vi "CAN-SET.vi"(6 "DevIndex":u32, 9 "open?":bool, 10 "type":u32(ring)=2 items=["USB-CAN"=2, "USB-CAN2.0"=3]) -> (2 "success":bool, 3 "Param out":T2[](array[typedef]) {"ACR0" format="%x"})   [LabVIEW 2011]
doc: "ID=0x6000"
uses:
  VIs/Param.ctl
  VIs/Baud rate Self Define.ctl
  VIs/ParamType.ctl
panel:
  out "label3":string="注：CAN波特率=16000000/(同步段+传播时间段+相位缓冲段1+相位缓冲段2)/预分频"
  out "label4":string="滤波器"
  out "label1":string="工作模式"
  out "label2":string="波特率设置"
  in  "advance":bool
  in  "br_selfdef":T1={"BAUD"=0, "SJW"=1, "BRP"=1, "SAM"=0, "PHS2_SEL"=0, "SYN(nouse)"=1, "PRSEG"=1, "PHSEG1"=1, "PHSEG2"=1} {"PHSEG2" items=["CAN_BIT_1TQ"=1, "CAN_BIT_2TQ"=2, "CAN_BIT_3TQ"=3, "CAN_BIT_4TQ"=4, "CAN_BIT_5TQ"=5, "CAN_BIT_6TQ"=6, "CAN_BIT_7TQ"=7, "CAN_BIT_8TQ"=8]; "PHSEG1" items=["CAN_BIT_1TQ"=1, "CAN_BIT_2TQ"=2, "CAN_BIT_3TQ"=3, "CAN_BIT_4TQ"=4, "CAN_BIT_5TQ"=5, "CAN_BIT_6TQ"=6, "CAN_BIT_7TQ"=7, "CAN_BIT_8TQ"=8]; "PRSEG" items=["CAN_BIT_1TQ"=1, "CAN_BIT_2TQ"=2, "CAN_BIT_3TQ"=3, "CAN_BIT_4TQ"=4, "CAN_BIT_5TQ"=5, "CAN_BIT_6TQ"=6, "CAN_BIT_7TQ"=7, "CAN_BIT_8TQ"=8]; "PHS2_SEL" items=["由相位缓冲段1时间指定", "可编程"]; "SAM" items=["采样一次", "采样三次"]; "BRP" items=["1"=1, "2"=2, "3"=3, "4"=4, "5"=5, "6"=6, "7"=7, "8"=8, "9"=9, "10"=10, "11"=11, "12"=12, "13"=13, "14"=14, "15"=15, "16"=16, "17"=17, "18"=18, "19"=19, "20"=20, "21"=21, "22"=22, "23"=23, "24"=24, "25"=25, "26"=26, "27"=27, "28"=28, "29"=29, "30"=30, "31"=31, "32"=32, "33"=33, "34"=34, "35"=35, "36"=36, "37"=37, "38"=38, "39"=39, "40"=40, "41"=41, "42"=42, "43"=43, "44"=44, "45"=45, "46"=46, "47"=47, "48"=48, "49"=49, "50"=50, "51"=51, "52"=52, "53"=53, "54"=54, "55"=55, "56"=56, "57"=57, "58"=58, "59"=59, "60"=60, "61"=61, "62"=62, "63"=63, "64"=64]; "SJW" items=["1TQ"=1, "2TQ"=2, "3TQ"=3, "4TQ"=4]; "SYN(nouse)" items=["CAN_BIT_1TQ"=1]}
  in  "Filter":u8(ring)=1 caption="滤波方式:" items=["接收所有类型"=1, "只收标准帧"=2, "只收扩展帧"=3]
  in  "set2":bool
  in  "set1":bool
  in  "channel":u16(ring) caption="CAN通道:" items=["通道1", "通道2"]
  in  "屏蔽码":u32=4294967295 caption="过滤屏蔽码:" format="%08x"
  in  "验收码":u32=2147483648 caption="过滤验收码:" format="%08x"
  in  "工作模式":u16(ring) items=["正常工作", "监听(只听)", "自发自收(环回/自测)", "正常工作并接收错误帧"]
  in  "set0":bool
  in  "br":u32(ring)=8 caption="波特率:" items=["Self Define", "5k bps", "10k bps", "20k bps", "40k bps", "50k bps", "80k bps", "100k bps", "125k bps", "200k bps", "250k bps", "400k bps", "500k bps", "666k bps", "800k bps", "1000k bps", "33.33k bps", "66.66k bps", "83.33k bps"]
  # "(HEX)"
  # "(HEX)"
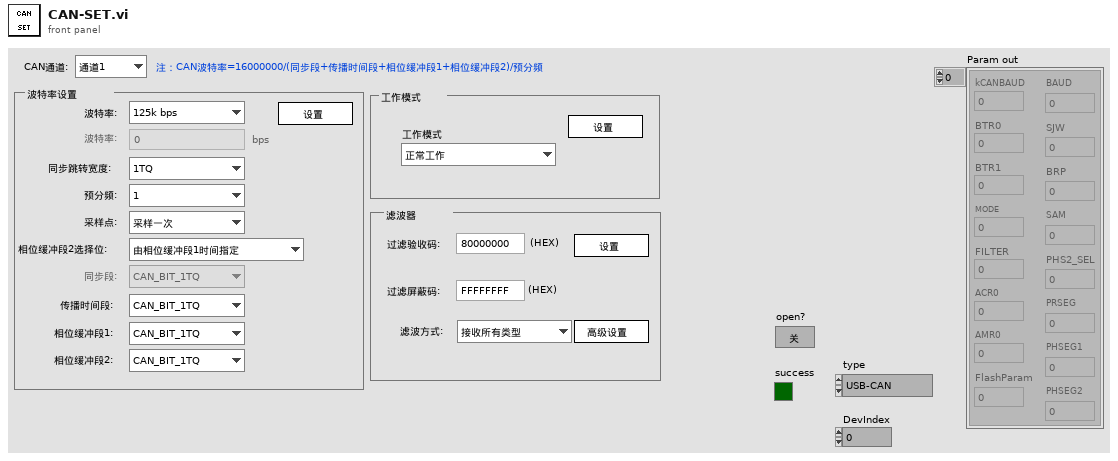
[diagram p1: front panel]
types:
  T1 = typedef "Baud rate Self Define.ctl" = cluster{"BAUD":u32, "SJW":u8, "BRP":u8, "SAM":u8, "PHS2_SEL":u8, "SYN(nouse)":u8, "PRSEG":u8, "PHSEG1":u8, "PHSEG2":u8}
  T2 = typedef "Param.ctl" = cluster{"kCANBAUD":u8, "BTR0":u8, "BTR1":u8, "MODE":u8, "FILTER":u8, "ACR0":u32, "AMR0":u32, "FlashParam":u32, "BAUD":u32, "SJW":u8, "BRP":u8, "SAM":u8, "PHS2_SEL":u8, "PRSEG":u8, "PHSEG1":u8, "PHSEG2":u8}
  T3 = enum8{"Enabled", "Disabled", "Disabled and Grayed Out"}
  T4 = typedef "ParamType.ctl" = u32
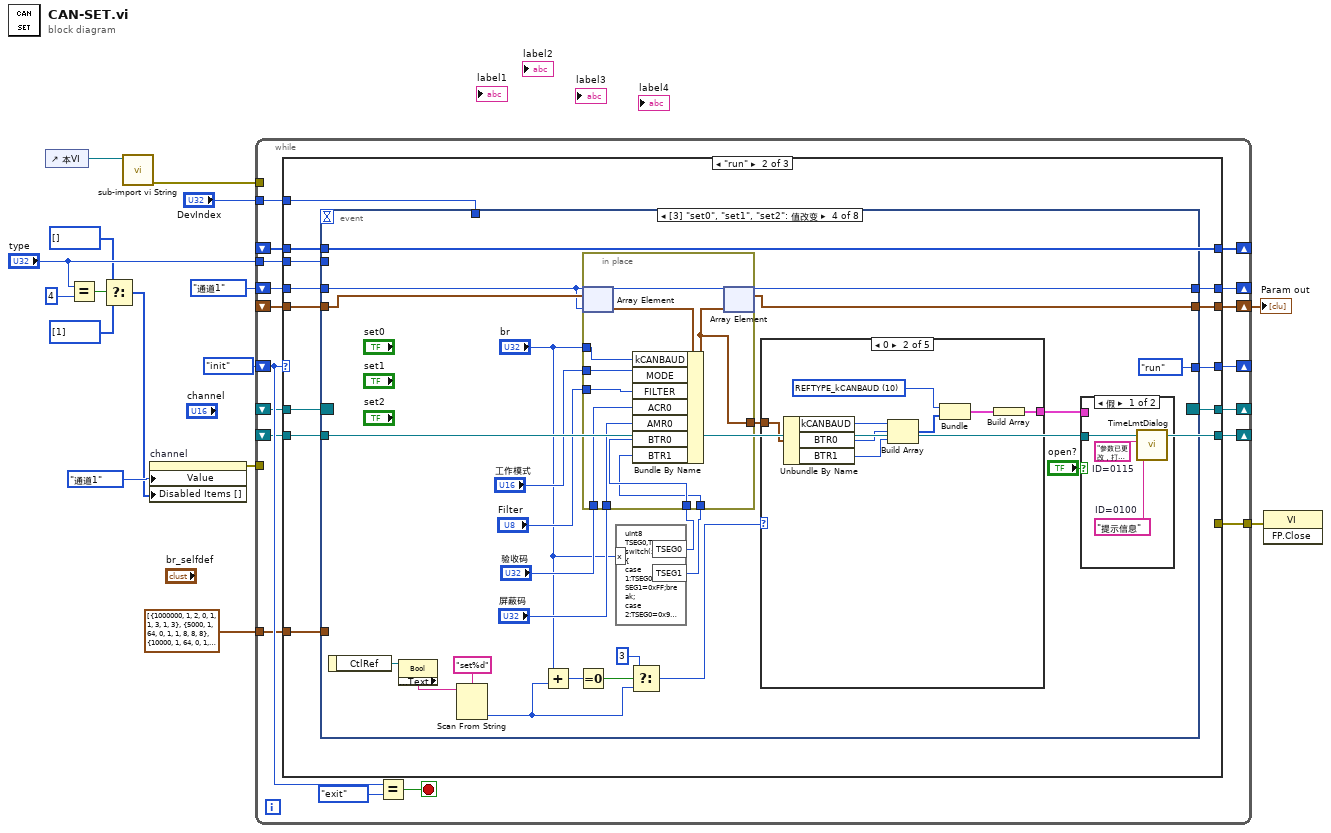
[diagram p0: block diagram]
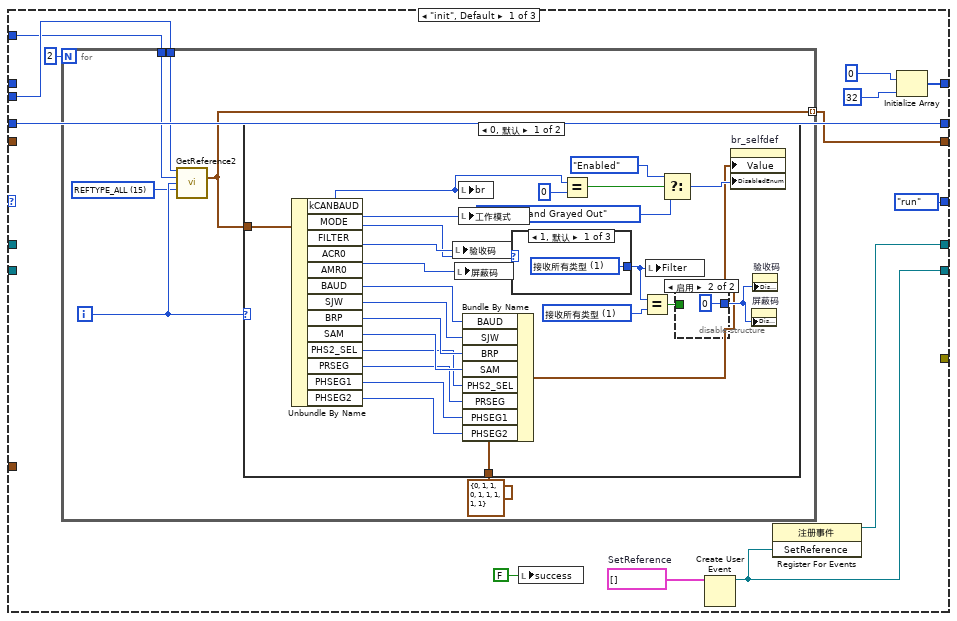
[diagram p2: hidden frame]
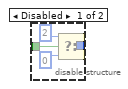
[diagram p3: hidden frame]
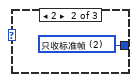
[diagram p4: hidden frame]
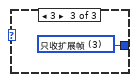
[diagram p5: hidden frame]
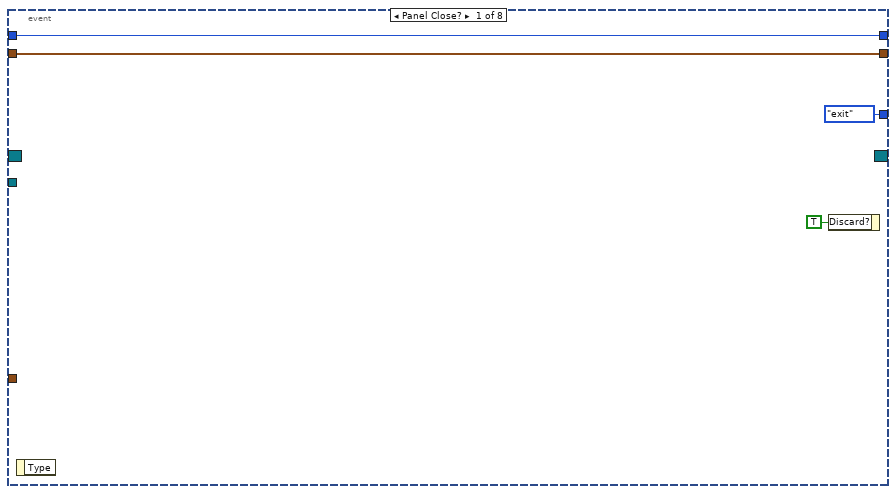
[diagram p7: hidden frame]
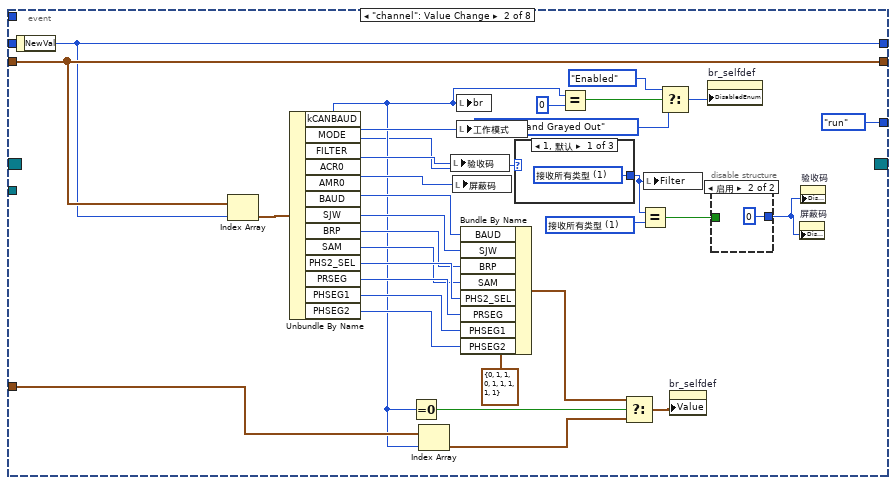
[diagram p8: hidden frame]
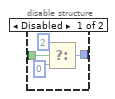
[diagram p9: hidden frame]
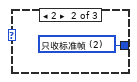
[diagram p10: hidden frame]
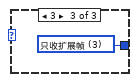
[diagram p11: hidden frame]
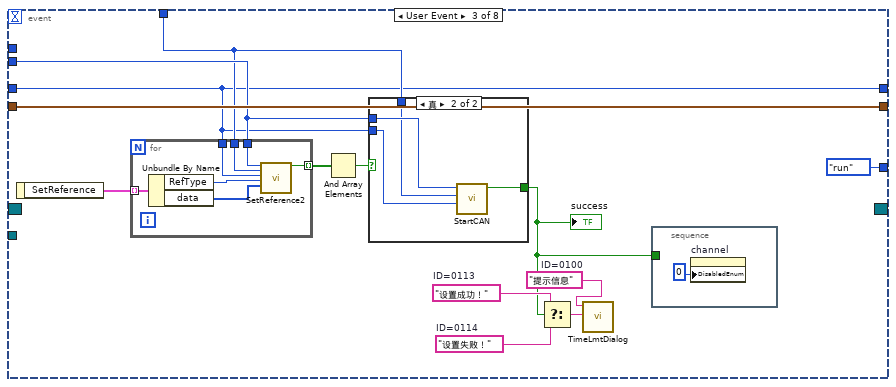
[diagram p12: hidden frame]
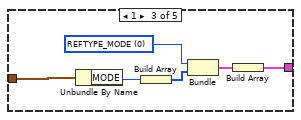
[diagram p15: hidden frame]
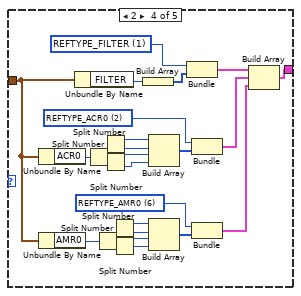
[diagram p16: hidden frame]
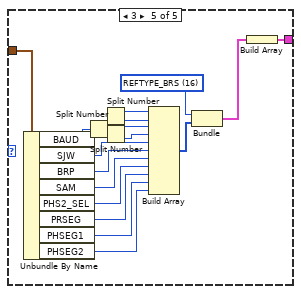
[diagram p17: hidden frame]
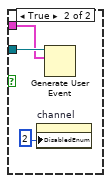
[diagram p18: hidden frame]
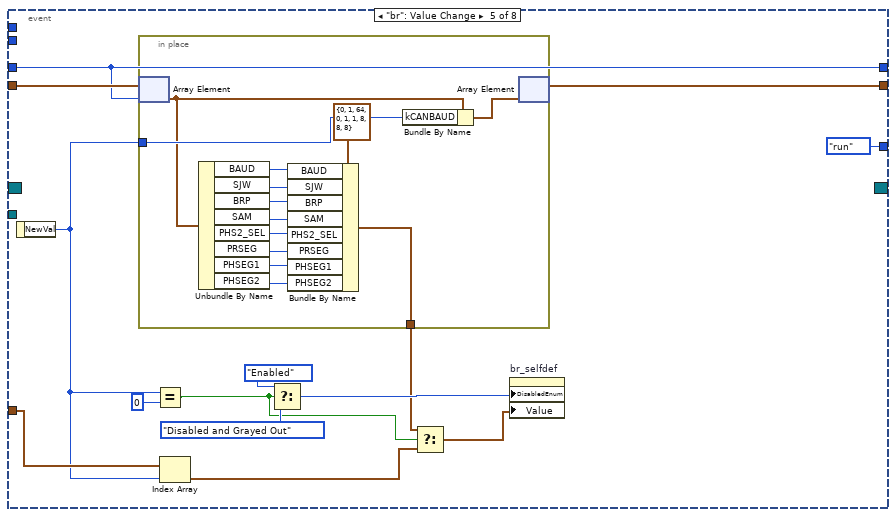
[diagram p19: hidden frame]
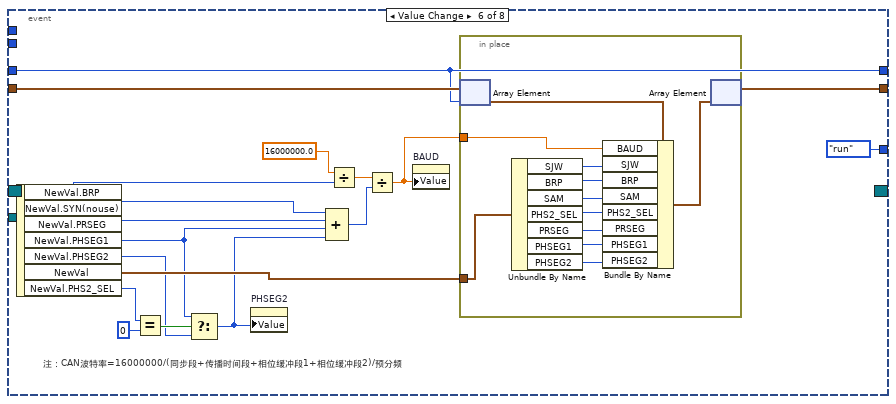
[diagram p20: hidden frame]
diagram:
  n1 = control-ref of="本VI"() -> (w2:refnum<vi>)
  n2 = Equal?(x="type", y=u32 4) -> (x = y?=w9:bool)
  n3 = Select(t=i32[] [] ("禁用项[]"), s=w9, f=i32[] [1] ("禁用项[]")) -> (s? t:f=w7:i32[])
  n4 = call "sub-import vi String.vi"("vi ref"=w2) -> ("error out"=w1:errorcluster)  [unwired: 10 in]
  n5 = property on="channel" class="Ring (严格)"("Value"=enum16{"通道1", "通道2"}."通道1" ("channel"), "Disabled Items []"=w7) -> (error out=w14:errorcluster)  [unwired: 2 in, 1 out]
  n6 = while {
    shift-right: [w33] -> w4
    shift-left: _ -> [w34]
    shift-right: [w32] -> _
    shift-left: enum16{"init", "run", "exit"}."init" -> [w31]
    tunnel: [w28] -> w15
    shift-right: [w27] -> _
    shift-left: _ -> [w25]
    shift-right: [w26] -> _
    shift-left: _ -> [w24]
    tunnel: "type" -> [w23]
    shift-right: [w22] -> _
    shift-left: _ -> [w21]
    tunnel: "DevIndex" -> [w20]
    shift-right: [w18] -> _
    shift-left: enum16{"通道1", "通道2"}."通道1" ("NewVal") -> [w19]
    tunnel: w14 -> [_]
    tunnel: T1[] [{"BAUD"=1000000, "SJW"=1, "BRP"=2, "SAM"=0, "PHS2_SEL"=1, "SYN(nouse)"=1, "PRSEG"=3, "PHSEG1"=1, "PHSEG2"=3}, {"BAUD"=5000, "SJW"=1, "BRP"=64, "SAM"=0, "PHS2_SEL"=1, "SYN(nouse)"=1, "PRSEG"=8, "PHSEG1"=8, "PHSEG2"=8}, {"BAUD"=10000, "SJW"=1, "BRP"=64, "SAM"=0, "PHS2_SEL"=1, "SYN(nouse)"=1, "PRSEG"=8, "PHSEG1"=8, "PHSEG2"=8}, {"BAUD"=20000, "SJW"=1, "BRP"=50, "SAM"=0, "PHS2_SEL"=1, "SYN(nouse)"=1, "PRSEG"=5, "PHSEG1"=5, "PHSEG2"=5}, {"BAUD"=40000, "SJW"=1, "BRP"=16, "SAM"=0, "PHS2_SEL"=1, "SYN(nouse)"=1, "PRSEG"=8, "PHSEG1"=8, "PHSEG2"=8}, {"BAUD"=50000, "SJW"=1, "BRP"=20, "SAM"=0, "PHS2_SEL"=1, "SYN(nouse)"=1, "PRSEG"=5, "PHSEG1"=5, "PHSEG2"=5}, {"BAUD"=80000, "SJW"=1, "BRP"=8, "SAM"=0, "PHS2_SEL"=1, "SYN(nouse)"=1, "PRSEG"=8, "PHSEG1"=8, "PHSEG2"=8}, {"BAUD"=100000, "SJW"=1, "BRP"=10, "SAM"=0, "PHS2_SEL"=1, "SYN(nouse)"=1, "PRSEG"=7, "PHSEG1"=4, "PHSEG2"=4}, {"BAUD"=125000, "SJW"=1, "BRP"=8, "SAM"=0, "PHS2_SEL"=1, "SYN(nouse)"=1, "PRSEG"=7, "PHSEG1"=4, "PHSEG2"=4}, {"BAUD"=200000, "SJW"=1, "BRP"=4, "SAM"=0, "PHS2_SEL"=1, "SYN(nouse)"=1, "PRSEG"=7, "PHSEG1"=6, "PHSEG2"=6}, {"BAUD"=250000, "SJW"=1, "BRP"=4, "SAM"=0, "PHS2_SEL"=1, "SYN(nouse)"=1, "PRSEG"=7, "PHSEG1"=4, "PHSEG2"=4}, {"BAUD"=400000, "SJW"=1, "BRP"=2, "SAM"=0, "PHS2_SEL"=1, "SYN(nouse)"=1, "PRSEG"=7, "PHSEG1"=6, "PHSEG2"=6}, {"BAUD"=500000, "SJW"=1, "BRP"=2, "SAM"=0, "PHS2_SEL"=1, "SYN(nouse)"=1, "PRSEG"=7, "PHSEG1"=4, "PHSEG2"=4}, {"BAUD"=666000, "SJW"=1, "BRP"=2, "SAM"=0, "PHS2_SEL"=1, "SYN(nouse)"=1, "PRSEG"=3, "PHSEG1"=4, "PHSEG2"=4}, {"BAUD"=800000, "SJW"=1, "BRP"=2, "SAM"=0, "PHS2_SEL"=1, "SYN(nouse)"=1, "PRSEG"=3, "PHSEG1"=3, "PHSEG2"=3}, {"BAUD"=1000000, "SJW"=1, "BRP"=2, "SAM"=0, "PHS2_SEL"=1, "SYN(nouse)"=1, "PRSEG"=3, "PHSEG1"=1, "PHSEG2"=3}, {"BAUD"=33333, "SJW"=1, "BRP"=32, "SAM"=0, "PHS2_SEL"=1, "SYN(nouse)"=1, "PRSEG"=4, "PHSEG1"=5, "PHSEG2"=5}, {"BAUD"=66666, "SJW"=1, "BRP"=16, "SAM"=0, "PHS2_SEL"=1, "SYN(nouse)"=1, "PRSEG"=4, "PHSEG1"=5, "PHSEG2"=5}, {"BAUD"=83333, "SJW"=1, "BRP"=8, "SAM"=0, "PHS2_SEL"=1, "SYN(nouse)"=1, "PRSEG"=7, "PHSEG1"=8, "PHSEG2"=8}] -> [w17]
    tunnel: w1 -> [_]
    stop <- w29 stop-if-true
    n7 = case shown="\"run\"" w31 {
      tunnel: w34 -> [_ w98 w370]
      tunnel: [w37 w97 w370] -> w33
      tunnel: [enum16{"init", "run", "exit"}."run" w96 enum16{"init", "run", "exit"}."exit"] -> w32
      tunnel: [_ _ errorcluster {"status"=FALSE, "code"=0, "source"=""} ("错误输入（无错误）")] -> w28
      tunnel: [w46 w91 _] -> w27
      tunnel: [w45 w92 _] -> w26
      tunnel: w25 -> [_ w95 w367]
      tunnel: w24 -> [_ w92 w365]
      tunnel: w23 -> [w36 w94 _]
      tunnel: [w42 w93 _] -> w22
      tunnel: w21 -> [_ w93 _]
      tunnel: w20 -> [w35 w90 _]
      tunnel: w19 -> [w39 w89 w364]
      tunnel: [w39 w88 w364] -> w18
      tunnel: w17 -> [_ w87 _]
      frame "init", Default {
        w40 = cluster{"RefType":u32, "data":u8[]}[] []  # SetReference
        n8 = for {
          N: 2 -> [_]
          tunnel: [w48] -> w37 mode=indexing
          tunnel: w36 -> [w52]
          tunnel: w35 -> [w51]
          i -> [w53]
          w50 = T4 15 items=["REFTYPE_MODE"=0, "REFTYPE_FILTER"=1, "REFTYPE_ACR0"=2, "REFTYPE_AMR0"=6, "REFTYPE_kCANBAUD"=10, "REFTYPE_CANRX_EN"=13, "REFTYPE_UARTBAUD"=14, "REFTYPE_ALL"=15, "REFTYPE_BRS"=16] ("RefType")
          n9 = call "GetReference2.vi"("DeviceType"=w52, "DeviceInd"=w51, "CANInd"=w53, "RefType"=w50) -> ("Param"=w48:T2)  [unwired: 9 in, 2 out]
          n10 = case shown="0, 默认" w53 {
            tunnel: w48 -> [w72 _]
            tunnel: T1 {"BAUD"=0, "SJW"=1, "BRP"=1, "SAM"=0, "PHS2_SEL"=1, "SYN(nouse)"=1, "PRSEG"=1, "PHSEG1"=1, "PHSEG2"=1} ("br_selfdef") -> [w69 _]
            frame 0, Default {
              w55 = u8 1 items=["接收所有类型"=1, "只收标准帧"=2, "只收扩展帧"=3] ("Filter")
              n11 = Unbundle By Name(w72) -> ("kCANBAUD"=w58:u8, "MODE"=w78:u8, "FILTER"=w56:u8, "ACR0"=w77:u32, "AMR0"=w76:u32, "BAUD"=w67:u32, "SJW"=w66:u8, "BRP"=w65:u8, "SAM"=w64:u8, "PHS2_SEL"=w63:u8, "PRSEG"=w62:u8, "PHSEG1"=w61:u8, "PHSEG2"=w60:u8)
              n12 = local write "验收码"(w77) -> ()
              n13 = local write "屏蔽码"(w76) -> ()
              n14 = local write "br"(w58) -> ()
              n15 = local write "工作模式"(w78) -> ()
              n16 = Bundle By Name(cluster=w69, "BAUD"=w67, "SJW"=w66, "BRP"=w65, "SAM"=w64, "PHS2_SEL"=w63, "PRSEG"=w62, "PHSEG1"=w61, "PHSEG2"=w60) -> (w57:T1)
              n17 = case shown="1, 默认" w56 {
                tunnel: [w84 w85 w86] -> w54
                frame 1, Default {
                  w84 = u8 1 items=["接收所有类型"=1, "只收标准帧"=2, "只收扩展帧"=3] ("Filter")
                }
                frame 2 {
                  w85 = u8 2 items=["接收所有类型"=1, "只收标准帧"=2, "只收扩展帧"=3] ("Filter")
                }
                frame 3 {
                  w86 = u8 3 items=["接收所有类型"=1, "只收标准帧"=2, "只收扩展帧"=3] ("Filter")
                }
              }
              n18 = Equal?(x=w58, y=u32 0) -> (x = y?=w59:bool)
              n19 = Equal?(x=w54, y=w55) -> (x = y?=w71:bool)
              n20 = local write "Filter"(w54) -> ()
              n21 = Select(t=T3."Enabled" ("禁用"), s=w59, f=T3."Disabled and Grayed Out") -> (s? t:f=w68:T3)
              n22 = disable-structure shown="启用" {
                disable-tunnel: w71 -> [w82 _]
                disable-tunnel: [w81 0] -> w70
                frame Disabled {
                  n23 = Select(t=2, s=w82, f=0) -> (s? t:f=w81:i32)
                }
                frame Enabled {
                }
              }
              n24 = property on="br_selfdef" class="Clust (严格)"("Value"=w57, "DisabledEnum"=w68) -> ()  [unwired: 2 in, 2 out]
              n25 = property on="屏蔽码" class="DigNum (严格)"("DisabledEnum"=w70) -> ()  [unwired: 2 in, 2 out]
              n26 = property on="验收码" class="DigNum (严格)"("DisabledEnum"=w70) -> ()  [unwired: 2 in, 2 out]
            }
            frame 1 {
            }
          }
        }
        n27 = local write "success"(FALSE ("success")) -> ()
        n28 = Create User Event(user event datatype=w40) -> (user event=w45:refnum<user-event>)  [unwired: 1 in, 1 out]
        n29 = register-events(w45) -> (reference out=w46:refnum<event-registration>)  [unwired: 2 in, 1 out]
        n30 = Initialize Array(u8 0, 32 ("维数大小")) -> (w42:u8[])
      }
      frame "run" {
        n31 = event shown="[3] \"set0\", \"set1\", \"set2\": 值改变" {
          selector: w95 -> [_ _ _ _ _ _ _ _]
          dyn-events: [_ _ _ _ _ _ _ _] -> w91
          timeout: _ -> [_ _ _ _ _ _ _ _]
          tunnel: w98 -> [w101 w133 w155 w180 w273 w302 w323 w355]
          tunnel: [w101 w133 w155 w178 w272 w300 w321 w355] -> w97
          tunnel: [enum16{"init", "run", "exit"}."exit" enum16{"init", "run", "exit"}."run" enum16{"init", "run", "exit"}."run" enum16{"init", "run", "exit"}."run" enum16{"init", "run", "exit"}."run" enum16{"init", "run", "exit"}."run" enum16{"init", "run", "exit"}."run" enum16{"init", "run", "exit"}."run"] -> w96
          tunnel: w92 -> [_ _ _ w189 _ _ _ _]
          tunnel: w94 -> [_ _ w149 _ _ _ _ _]
          tunnel: w93 -> [_ _ _ _ _ _ _ _]
          tunnel: w90 -> [_ _ w148 _ _ _ _ _]
          tunnel: w89 -> [w99 _ w145 w179 w267 w301 w322 w358]
          tunnel: [w99 w132 w145 w179 w267 w301 w322 w358] -> w88
          tunnel: w87 -> [_ w108 _ _ w268 _ _ _]
          event Panel Close? {
            n32 = event-data() -> ()  [unwired: 1 in, 1 out]
            n33 = event-data("Discard?"=TRUE ("放弃？")) -> ()  [unwired: 1 in, 1 out]
          }
          event "channel": Value Change {
            w103 = u8 1 items=["接收所有类型"=1, "只收标准帧"=2, "只收扩展帧"=3] ("Filter")
            n34 = event-data() -> ("NewVal"=w132:u16)  [unwired: 1 in]
            n35 = Index Array(array=w133, index=w132) -> (element=w112:T2)
            n36 = Unbundle By Name(w112) -> ("kCANBAUD"=w107:u8, "MODE"=w114:u8, "FILTER"=w105:u8, "ACR0"=w115:u32, "AMR0"=w116:u32, "BAUD"=w123:u32, "SJW"=w124:u8, "BRP"=w125:u8, "SAM"=w126:u8, "PHS2_SEL"=w127:u8, "PRSEG"=w128:u8, "PHSEG1"=w129:u8, "PHSEG2"=w130:u8)
            n37 = Equal To 0?(x=w107) -> (x = 0?=w111:bool)
            n38 = Index Array(array=w108, index=w107) -> (element=w106:T1)
            n39 = local write "验收码"(w115) -> ()
            n40 = local write "屏蔽码"(w116) -> ()
            n41 = local write "br"(w107) -> ()
            n42 = local write "工作模式"(w114) -> ()
            n43 = Bundle By Name(cluster=T1 {"BAUD"=0, "SJW"=1, "BRP"=1, "SAM"=0, "PHS2_SEL"=1, "SYN(nouse)"=1, "PRSEG"=1, "PHSEG1"=1, "PHSEG2"=1} ("br_selfdef"), "BAUD"=w123, "SJW"=w124, "BRP"=w125, "SAM"=w126, "PHS2_SEL"=w127, "PRSEG"=w128, "PHSEG1"=w129, "PHSEG2"=w130) -> (w110:T1)
            n44 = case shown="1, 默认" w105 {
              tunnel: [w140 w141 w142] -> w104
              frame 1, Default {
                w140 = u8 1 items=["接收所有类型"=1, "只收标准帧"=2, "只收扩展帧"=3] ("Filter")
              }
              frame 2 {
                w141 = u8 2 items=["接收所有类型"=1, "只收标准帧"=2, "只收扩展帧"=3] ("Filter")
              }
              frame 3 {
                w142 = u8 3 items=["接收所有类型"=1, "只收标准帧"=2, "只收扩展帧"=3] ("Filter")
              }
            }
            n45 = Equal?(x=w107, y=u32 0) -> (x = y?=w131:bool)
            n46 = Select(t=w110, s=w111, f=w106) -> (s? t:f=w109:T1)
            n47 = Equal?(x=w104, y=w103) -> (x = y?=w120:bool)
            n48 = local write "Filter"(w104) -> ()
            n49 = Select(t=T3."Enabled" ("禁用"), s=w131, f=T3."Disabled and Grayed Out") -> (s? t:f=w122:T3)
            n50 = property on="br_selfdef" class="Clust (严格)"("Value"=w109) -> ()  [unwired: 2 in, 2 out]
            n51 = property on="br_selfdef" class="Clust (严格)"("DisabledEnum"=w122) -> ()  [unwired: 2 in, 2 out]
            n52 = disable-structure shown="启用" {
              disable-tunnel: [w136 0] -> w121
              disable-tunnel: w120 -> [w135 _]
              frame Disabled {
                n53 = Select(t=2, s=w135, f=0) -> (s? t:f=w136:i32)
              }
              frame Enabled {
              }
            }
            n54 = property on="屏蔽码" class="DigNum (严格)"("DisabledEnum"=w121) -> ()  [unwired: 2 in, 2 out]
            n55 = property on="验收码" class="DigNum (严格)"("DisabledEnum"=w121) -> ()  [unwired: 2 in, 2 out]
          }
          event User Event {
            w143 = "提示信息"  # ID=0100
            w152 = "设置失败！"  # ID=0114
            w153 = "设置成功！"  # ID=0113
            n56 = event-data() -> ("SetReference"=w147:cluster{"RefType":u32, "data":u8[]}[])  [unwired: 1 in]
            n57 = for {
              tunnel: [w163] -> w150 mode=indexing
              tunnel: w149 -> [w162]
              tunnel: w148 -> [w161]
              tunnel: w145 -> [w160]
              tunnel: w147 -> [w159] mode=indexing
              n58 = Unbundle By Name(w159) -> ("RefType"=w158:u32, "data"=w157:u8[])
              n59 = call "SetReference2.vi"("DeviceType"=w162, "DeviceInd"=w161, "CANInd"=w160, "RefType"=w158, "pData"=w157) -> ("Success"=w163:bool)  [unwired: 13 in, 1 out]
            }
            n60 = And Array Elements(Boolean array=w150) -> (logical AND=w146:bool)
            n61 = case shown="真" w146 {
              tunnel: w149 -> [_ w167]
              tunnel: w145 -> [_ w165]
              tunnel: [_ w164] -> w144
              tunnel: w148 -> [_ w166]
              frame False {
              }
              frame True {
                n62 = call "StartCAN.vi"("CANInd"=w165, "DeciceInd"=w166, "DeviceType"=w167) -> ("Valid"=w164:bool)  [unwired: 7 in, 1 out]
              }
            }
            "success" <- w144
            n63 = Select(t=w153, s=w144, f=w152) -> (s? t:f=w151:string)
            n64 = call "TimeLmtDialog.vi"("Infoin"=w151, "title"=w143) -> ()  [unwired: 10 in]
            n65 = stacked-sequence {
              tunnel: w144 -> [_]
              frame #0 {
                n66 = property on="channel" class="Ring (严格)"("DisabledEnum"=0) -> ()  [unwired: 2 in, 2 out]
              }
            }
          }
          event "set0", "set1", "set2": Value Change {
            n67 = event-data() -> ("CtlRef"=w184:refnum<vi>)  [unwired: 1 in]
            n68 = property class="Bool"(reference=w184) -> ("Label.Text"=w183:string)  [unwired: 1 in, 2 out]
            n69 = Scan From String(format string="set%d" ("格式字符串"), input string=w183) -> (output 1=w173:i32)  [unwired: 3 in, 3 out]
            n70 = Add(x="br", y=w173) -> (x+y=w172:u32)
            n71 = Equal To 0?(x=w172) -> (x = 0?=w171:bool)
            n72 = formula code="uInt8 TSEG0,TSEG1;\nswitch(x)\n{ \ncase 1:TSEG0=0x9F;TSEG1=0xFF;break;\ncase 2:TSEG0=0x9F;TSEG1=0xFF;break;\ncase 3:TSEG0=0x18;TSEG1=0x1c;break;\ncase 4:TSEG0=0x87;TSEG1=0xff;break;\ncase 5:TSEG0=0x09;TSEG1=0x1c;break;\ncase 6:TSEG0=0x83;TSEG1=0xff;break;\ncase 7:TSEG0=0x04;TSEG1=0x1c;break;\ncase 8:TSEG0=0x03;TSEG1=0x1c;break;\ncase 9:TSEG0=0x81;TSEG1=0xfa;break;\ncase 10:TSEG0=0x01;TSEG1=0x1c;break;\ncase 11:TSEG0=0x80;TSEG1=0xfa;break;\ncase 12:TSEG0=0x00;TSEG1=0x1c;break;\ncase 13:TSEG0=0x80;TSEG1=0xb6;break;\ncase 14:TSEG0=0x00;TSEG1=0x16;break;\ncase 15:TSEG0=0x00;TSEG1=0x14;break;\ncase 16:TSEG0=0x09;TSEG1=0x6F;break;\ncase 17:TSEG0=0x04;TSEG1=0x6F;break;\ncase 18:TSEG0=0x03;TSEG1=0x6F;break;\ndefault:break;\n}"("x"="br") -> ("TSEG0"=w169:u8, "TSEG1"=w168:u8)
            n73 = in-place {
              in-place-border: "br" -> [w199]
              in-place-border: "工作模式" -> [w198]
              in-place-border: "验收码" -> [w197]
              in-place-border: "屏蔽码" -> [w196]
              in-place-border: [w194] -> w177
              in-place-border: "Filter" -> [w193]
              in-place-border: w169 -> [w192]
              in-place-border: w168 -> [w191]
              n74 = in-place-array #1(w180, w179) -> (w195:T2)
              n75 = Bundle By Name(cluster=w195, "kCANBAUD"=w199, "MODE"=w198, "FILTER"=w193, "ACR0"=w197, "AMR0"=w196, "BTR0"=w192, "BTR1"=w191) -> (w194:T2)
              n76 = in-place-array #1(w194) -> (w178:T2[])  [unwired: 1 out]
            }
            n77 = Select(t=3, s=w171, f=w173) -> (s? t:f=w174:i32)
            n78 = case shown="0" w174 {
              tunnel: w177 -> [_ w207 w213 w221 w250]
              tunnel: [_ w201 w209 w217 w249] -> w181
              frame -1, Default {
              }
              frame 0 {
                w200 = T4 10 items=["REFTYPE_MODE"=0, "REFTYPE_FILTER"=1, "REFTYPE_ACR0"=2, "REFTYPE_AMR0"=6, "REFTYPE_kCANBAUD"=10, "REFTYPE_CANRX_EN"=13, "REFTYPE_UARTBAUD"=14, "REFTYPE_ALL"=15, "REFTYPE_BRS"=16] ("RefType")
                n79 = Unbundle By Name(w207) -> ("kCANBAUD"=w206:u8, "BTR0"=w205:u8, "BTR1"=w204:u8)
                n80 = Build Array(w206, w205, w204) -> (w203:u8[])
                n81 = Bundle("RefType"=w200, w203) -> (w202:cluster{"RefType":T4, u8[]})  [unwired: 1 in]
                n82 = Build Array(w202) -> (w201:cluster{"RefType":T4, u8[]}[])
              }
              frame 1 {
                w208 = T4 0 items=["REFTYPE_MODE"=0, "REFTYPE_FILTER"=1, "REFTYPE_ACR0"=2, "REFTYPE_AMR0"=6, "REFTYPE_kCANBAUD"=10, "REFTYPE_CANRX_EN"=13, "REFTYPE_UARTBAUD"=14, "REFTYPE_ALL"=15, "REFTYPE_BRS"=16] ("RefType")
                n83 = Unbundle By Name(w213) -> ("MODE"=w212:u8)
                n84 = Build Array(w212) -> (w211:u8[])
                n85 = Bundle("RefType"=w208, w211) -> (w210:cluster{"RefType":T4, u8[]})  [unwired: 1 in]
                n86 = Build Array(w210) -> (w209:cluster{"RefType":T4, u8[]}[])
              }
              frame 2 {
                w214 = T4 6 items=["REFTYPE_MODE"=0, "REFTYPE_FILTER"=1, "REFTYPE_ACR0"=2, "REFTYPE_AMR0"=6, "REFTYPE_kCANBAUD"=10, "REFTYPE_CANRX_EN"=13, "REFTYPE_UARTBAUD"=14, "REFTYPE_ALL"=15, "REFTYPE_BRS"=16] ("RefType")
                w215 = T4 2 items=["REFTYPE_MODE"=0, "REFTYPE_FILTER"=1, "REFTYPE_ACR0"=2, "REFTYPE_AMR0"=6, "REFTYPE_kCANBAUD"=10, "REFTYPE_CANRX_EN"=13, "REFTYPE_UARTBAUD"=14, "REFTYPE_ALL"=15, "REFTYPE_BRS"=16] ("RefType")
                w216 = T4 1 items=["REFTYPE_MODE"=0, "REFTYPE_FILTER"=1, "REFTYPE_ACR0"=2, "REFTYPE_AMR0"=6, "REFTYPE_kCANBAUD"=10, "REFTYPE_CANRX_EN"=13, "REFTYPE_UARTBAUD"=14, "REFTYPE_ALL"=15, "REFTYPE_BRS"=16] ("RefType")
                n87 = Unbundle By Name(w221) -> ("ACR0"=w236:u32)
                n88 = Unbundle By Name(w221) -> ("AMR0"=w223:u32)
                n89 = Unbundle By Name(w221) -> ("FILTER"=w239:u8)
                n90 = Split Number(x=w236) -> (hi(x)=w235:u16, lo(x)=w234:u16)
                n91 = Split Number(x=w223) -> (hi(x)=w224:u16, lo(x)=w225:u16)
                n92 = Split Number(x=w235) -> (hi(x)=w233:u8, lo(x)=w232:u8)
                n93 = Split Number(x=w234) -> (hi(x)=w231:u8, lo(x)=w230:u8)
                n94 = Split Number(x=w224) -> (hi(x)=w226:u8, lo(x)=w227:u8)
                n95 = Split Number(x=w225) -> (hi(x)=w228:u8, lo(x)=w229:u8)
                n96 = Build Array(w239) -> (w238:u8[])
                n97 = Build Array(w233, w232, w231, w230) -> (w237:u8[])
                n98 = Build Array(w226, w227, w228, w229) -> (w222:u8[])
                n99 = Bundle("RefType"=w216, w238) -> (w220:cluster{"RefType":T4, u8[]})  [unwired: 1 in]
                n100 = Bundle("RefType"=w215, w237) -> (w219:cluster{"RefType":T4, u8[]})  [unwired: 1 in]
                n101 = Bundle("RefType"=w214, w222) -> (w218:cluster{"RefType":T4, u8[]})  [unwired: 1 in]
                n102 = Build Array(w220, w219, w218) -> (w217:cluster{"RefType":T4, u8[]}[])
              }
              frame 3 {
                w247 = T4 16 items=["REFTYPE_MODE"=0, "REFTYPE_FILTER"=1, "REFTYPE_ACR0"=2, "REFTYPE_AMR0"=6, "REFTYPE_kCANBAUD"=10, "REFTYPE_CANRX_EN"=13, "REFTYPE_UARTBAUD"=14, "REFTYPE_ALL"=15, "REFTYPE_BRS"=16] ("RefType")
                n103 = Unbundle By Name(w250) -> ("BAUD"=w257:u32, "SJW"=w246:u8, "BRP"=w245:u8, "SAM"=w244:u8, "PHS2_SEL"=w243:u8, "PRSEG"=w242:u8, "PHSEG1"=w241:u8, "PHSEG2"=w240:u8)
                n104 = Split Number(x=w257) -> (hi(x)=w256:u16, lo(x)=w255:u16)
                n105 = Split Number(x=w256) -> (hi(x)=w254:u8, lo(x)=w253:u8)
                n106 = Split Number(x=w255) -> (hi(x)=w252:u8, lo(x)=w251:u8)
                n107 = Build Array(w254, w253, w252, w251, w246, w245, w244, w243, w242, w241, w240) -> (w258:u8[])
                n108 = Bundle("RefType"=w247, w258) -> (w248:cluster{"RefType":T4, u8[]})  [unwired: 1 in]
                n109 = Build Array(w248) -> (w249:cluster{"RefType":T4, u8[]}[])
              }
            }
            n110 = case shown="假" "open?" {
              tunnel: w189 -> [_ w263]
              tunnel: w181 -> [_ w262]
              frame False {
                w259 = "提示信息"  # ID=0100
                w260 = "参数已更改，打开设备生效！"  # ID=0115
                n111 = call "TimeLmtDialog.vi"("Infoin"=w260, "title"=w259) -> ()  [unwired: 10 in]
              }
              frame True {
                n112 = property on="channel" class="Ring (严格)"("DisabledEnum"=2) -> ()  [unwired: 2 in, 2 out]
                n113 = Generate User Event(user event=w263, event data cluster=w262) -> ()  [unwired: 1 in, 2 out]
              }
            }
          }
          event "br": Value Change {
            n114 = event-data() -> ("NewVal"=w264:u32)  [unwired: 1 in]
            n115 = in-place {
              in-place-border: w264 -> [w290]
              in-place-border: [w278] -> w269
              n116 = in-place-array #2(w273, w267) -> (w288:T2)
              n117 = Unbundle By Name(w288) -> ("BAUD"=w279:u32, "SJW"=w280:u8, "BRP"=w281:u8, "SAM"=w282:u8, "PHS2_SEL"=w283:u8, "PRSEG"=w284:u8, "PHSEG1"=w285:u8, "PHSEG2"=w286:u8)
              n118 = Bundle By Name(cluster=T1 {"BAUD"=0, "SJW"=1, "BRP"=64, "SAM"=0, "PHS2_SEL"=1, "SYN(nouse)"=1, "PRSEG"=8, "PHSEG1"=8, "PHSEG2"=8} ("br_selfdef"), "BAUD"=w279, "SJW"=w280, "BRP"=w281, "SAM"=w282, "PHS2_SEL"=w283, "PRSEG"=w284, "PHSEG1"=w285, "PHSEG2"=w286) -> (w278:T1)
              n119 = Bundle By Name(cluster=w288, "kCANBAUD"=w290) -> (w289:T2)
              n120 = in-place-array #2(w289) -> (w272:T2[])  [unwired: 1 out]
            }
            n121 = Equal?(x=w264, y=u32 0) -> (x = y?=w270:bool)
            n122 = Index Array(array=w268, index=w264) -> (element=w266:T1)
            n123 = Select(t=T3."Enabled" ("禁用"), s=w270, f=T3."Disabled and Grayed Out") -> (s? t:f=w271:T3)
            n124 = Select(t=w269, s=w270, f=w266) -> (s? t:f=w265:T1)
            n125 = property on="br_selfdef" class="Clust (严格)"("DisabledEnum"=w271, "Value"=w265) -> ()  [unwired: 2 in, 2 out]
          }
          event Value Change {
            # "注：CAN波特率=16000000/(同步段+传播时间段+相位缓冲段1+相位缓冲段2)/预分频"
            n126 = event-data() -> ("NewVal.BRP"=w305:u8, "NewVal.SYN(nouse)"=w307:u8, "NewVal.PRSEG"=w294:u8, "NewVal.PHSEG1"=w291:u8, "NewVal.PHSEG2"=w293:u8, "NewVal"=w298:T1, "NewVal.PHS2_SEL"=w297:u8)  [unwired: 1 in]
            n127 = Equal?(x=w297, y=u8 0) -> (x = y?=w295:bool)
            n128 = Select(t=w291, s=w295, f=w293) -> (s? t:f=w292:u8)
            n129 = property on="PHSEG2" class="Ring (严格)"("Value"=w292) -> ()  [unwired: 2 in, 2 out]
            n130 = Compound Arithmetic op=ADD(w307, w294, w291, w292) -> (w303:u8)
            n131 = Divide(x=16000000.0, y=w305) -> (x/y=w304:dbl)
            n132 = Divide(x=w304, y=w303) -> (x/y=w299:dbl)
            n133 = property on="BAUD" class="DigNum (严格)"("Value"=w299) -> ()  [unwired: 2 in, 2 out]
            n134 = in-place {
              in-place-border: w299 -> [w317]
              in-place-border: w298 -> [w316]
              n135 = in-place-array #3(w302, w301) -> (w319:T2)
              n136 = Unbundle By Name(w316) -> ("SJW"=w309:u8, "BRP"=w310:u8, "SAM"=w311:u8, "PHS2_SEL"=w312:u8, "PRSEG"=w313:u8, "PHSEG1"=w314:u8, "PHSEG2"=w315:u8)
              n137 = Bundle By Name(cluster=w319, "BAUD"=w317, "SJW"=w309, "BRP"=w310, "SAM"=w311, "PHS2_SEL"=w312, "PRSEG"=w313, "PHSEG1"=w314, "PHSEG2"=w315) -> (w318:T2)
              n138 = in-place-array #3(w318) -> (w300:T2[])  [unwired: 1 out]
            }
          }
          event "Filter": Value Change {
            n139 = event-data() -> ("NewVal"=w320:u8)  [unwired: 1 in]
            n140 = in-place {
              in-place-border: w320 -> [w332]
              w333 = u8 1 items=["接收所有类型"=1, "只收标准帧"=2, "只收扩展帧"=3] ("Filter")
              n141 = in-place-array #4(w323, w322) -> (w329:T2)
              n142 = case shown="3" w332 {
                tunnel: [w347 w348 w349] -> w330
                frame 1, Default {
                  w347 = u8 1 items=["接收所有类型"=1, "只收标准帧"=2, "只收扩展帧"=3] ("Filter")
                }
                frame 2 {
                  w348 = u8 2 items=["接收所有类型"=1, "只收标准帧"=2, "只收扩展帧"=3] ("Filter")
                }
                frame 3 {
                  w349 = u8 3 items=["接收所有类型"=1, "只收标准帧"=2, "只收扩展帧"=3] ("Filter")
                }
              }
              n143 = Unbundle By Name(w329) -> ("ACR0"=w328:u32, "AMR0"=w327:u32)
              n144 = Equal?(x=w330, y=w333) -> (x = y?=w334:bool)
              n145 = local write "Filter"(w330) -> ()
              n146 = disable-structure shown="启用" {
                disable-tunnel: w334 -> [w343 _]
                disable-tunnel: w328 -> [w338 w346]
                disable-tunnel: w327 -> [w337 w345]
                disable-tunnel: [w336 w346] -> w326
                disable-tunnel: [w335 w345] -> w325
                frame Disabled {
                  n147 = Select(t=0, s=w343, f=0) -> (s? t:f=w339:i32)
                  n148 = Select(t=u32 0, s=w343, f=w338) -> (s? t:f=w336:u32)
                  n149 = Select(t=u32 4294967295, s=w343, f=w337) -> (s? t:f=w335:u32)
                  n150 = property on="屏蔽码" class="DigNum (严格)"("DisabledEnum"=w339, "Value"=w335) -> ()  [unwired: 2 in, 2 out]
                  n151 = property on="验收码" class="DigNum (严格)"("DisabledEnum"=w339, "Value"=w336) -> ()  [unwired: 2 in, 2 out]
                }
                frame Enabled {
                }
              }
              n152 = Bundle By Name(cluster=w329, "FILTER"=w330, "ACR0"=w326, "AMR0"=w325) -> (w331:T2)
              n153 = in-place-array #4(w331) -> (w321:T2[])  [unwired: 1 out]
            }
          }
          event "advance": Value Change {
            n154 = event-data() -> ()  [unwired: 1 in, 1 out]
            n155 = local read "验收码"() -> (w353:u32)
            n156 = local read "屏蔽码"() -> (w352:u32)
            n157 = local read "Filter"() -> (w354:u8)
            n158 = Bundle By Name(cluster=cluster{"mode":u8, "AccCode":u32, "AccMask":u32} {"mode"=1, "AccCode"=0, "AccMask"=4294967295} ("ParamIn"), "mode"=w354, "AccCode"=w353, "AccMask"=w352) -> (w356:cluster{"mode":u8, "AccCode":u32, "AccMask":u32})
            n159 = call "FilterSet.vi"("ParamIn"=w356) -> ("Cancel？"=w351:bool, "ParamOut"=w350:cluster{"mode":u8, "AccCode":u32, "AccMask":u32})  [unwired: 8 in, 1 out]
            n160 = case shown="假" w351 {
              tunnel: w350 -> [w363 _]
              frame False {
                n161 = Unbundle By Name(w363) -> ("mode"=w362:u8, "AccCode"=w361:u32, "AccMask"=w360:u32)
                n162 = local write "验收码"(w361) -> ()
                n163 = local write "屏蔽码"(w360) -> ()
                n164 = local write "Filter"(w362) -> ()
              }
              frame True {
              }
            }
          }
        }
      }
      frame "exit" {
        n165 = Unregister For Events(event registration refnum=w367) -> (error out=w366:errorcluster)  [unwired: 1 in]
        n166 = Destroy User Event(user event=w365, error in=w366) -> ()  [unwired: 1 out]
      }
    }
    n167 = Equal?(x=w31, y=enum16{"init", "run", "exit"}."exit") -> (x = y?=w29:bool)
  }
  "Param out" <- w4
  n168 = invoke class="VI" method="FP.Close"(error in=w15) -> ()  [unwired: 2 in, 3 out]
